vi "Vision Processing.vi"(4 "error in (no error)":errorcluster, 7 "Image Size":T1=enum."320x240") -> ()   [LabVIEW 2014]
uses:
  Vision Support Code/Camera Types.ctl
  <vilib>/Rock Robotics/WPI/Camera/WPI_CameraImageSize.ctl
  <vilib>/Rock Robotics/WPI/Camera/WPI_CameraWhite Balance Values.ctl
  <vilib>/Rock Robotics/WPI/Camera/WPI_CameraExposure Values.ctl
  <vilib>/Rock Robotics/WPI/Camera/WPI_CameraFrameRate.ctl
  Robot Global Data.vi
  <vilib>/vision/NI_Vision_Development_Module.lvlib
panel:
  in  "FPS":dbl
  out "Position_Debugger":i32
  in  "Right Boundary":dbl
  in  "Left Boundary":dbl
  out "Centering Command":enum16{"NULL", "RIGHT", "LEFT", "CENTER"}(ring)
  out "Horizontal Centering":dbl
  in  "Limit Tests?":bool
  in  "Camera Type":T2=enum."MS HD3000 square"
  in  "Aspect Fudge Factor":dbl=1.0
  out "Detected Totes":T3(array[cluster]) {"Normalized Rect"."Numeric 5" format="%#_2g"; "Normalized Rect"."Numeric 3" format="%#_2g"; "Normalized Rect"."Numeric 2" format="%#_2g"; "Normalized Rect"."Numeric" format="%#_2g"}
  in  "Score Threshold":dbl=75.0
  in  "Show Carpet Mask":bool
  in  "Carpet Color":T4(tab)
  in  "Red":T5={"Hue"={231.0, 14.0}, "Sat"={83.0, 255.0}, "Val"={52.5, 255.0}} {"Hue" scale=0.0..255.0 scale format="%#_3g"}
  in  "Blue":T5={"Hue"={119.0, 181.0}, "Sat"={33.0, 255.0}, "Val"={48.571428571428584, 255.0}} {"Hue" scale=0.0..255.0 scale format="%#_3g"}
  in  "Annotate":bool
  out "ms to process":u32
  out "Sorted Scores":T6(array[cluster]) {"Carpet" format="%#_3g"; "S" format="%#_3g"; "Trapezoid %" format="%#_3g"; "L" format="%#_3g"; "Area to CH" format="%#_3g"; "X" format="%#_3g"; "Y" format="%#_3g"}
  out "Particles":i32
  in  "Tote Color":T5={"Hue"={36.0, 50.923317529462665}, "Sat"={196.28571428571428, 255.0}, "Val"={163.92857142857144, 255.0}} {"Hue" scale=0.0..255.0 scale format="%#_3g"}
  out "Masked":T7(plugin-control)
  out "Original Image":T7(plugin-control)
  # "This is only the initial camera size.\nOther camera setup is done\non the diagram. Notice it is set\nonce before the loop but can be\nupdated within the loop if needed."
  # "Instructions:\nUse Source select image files from a directory or use a USB or IP camera connected to your laptop.\nUse Tote Color to threshold and build particles. Adjust calibration if needed.\nSelect which carpet color to use for scoring. Calibrate the colors if needed.\nAnnotations show the rectangle and the scores from top to bottom."
  # "Aspect Ratio"
  # "Density Profile"
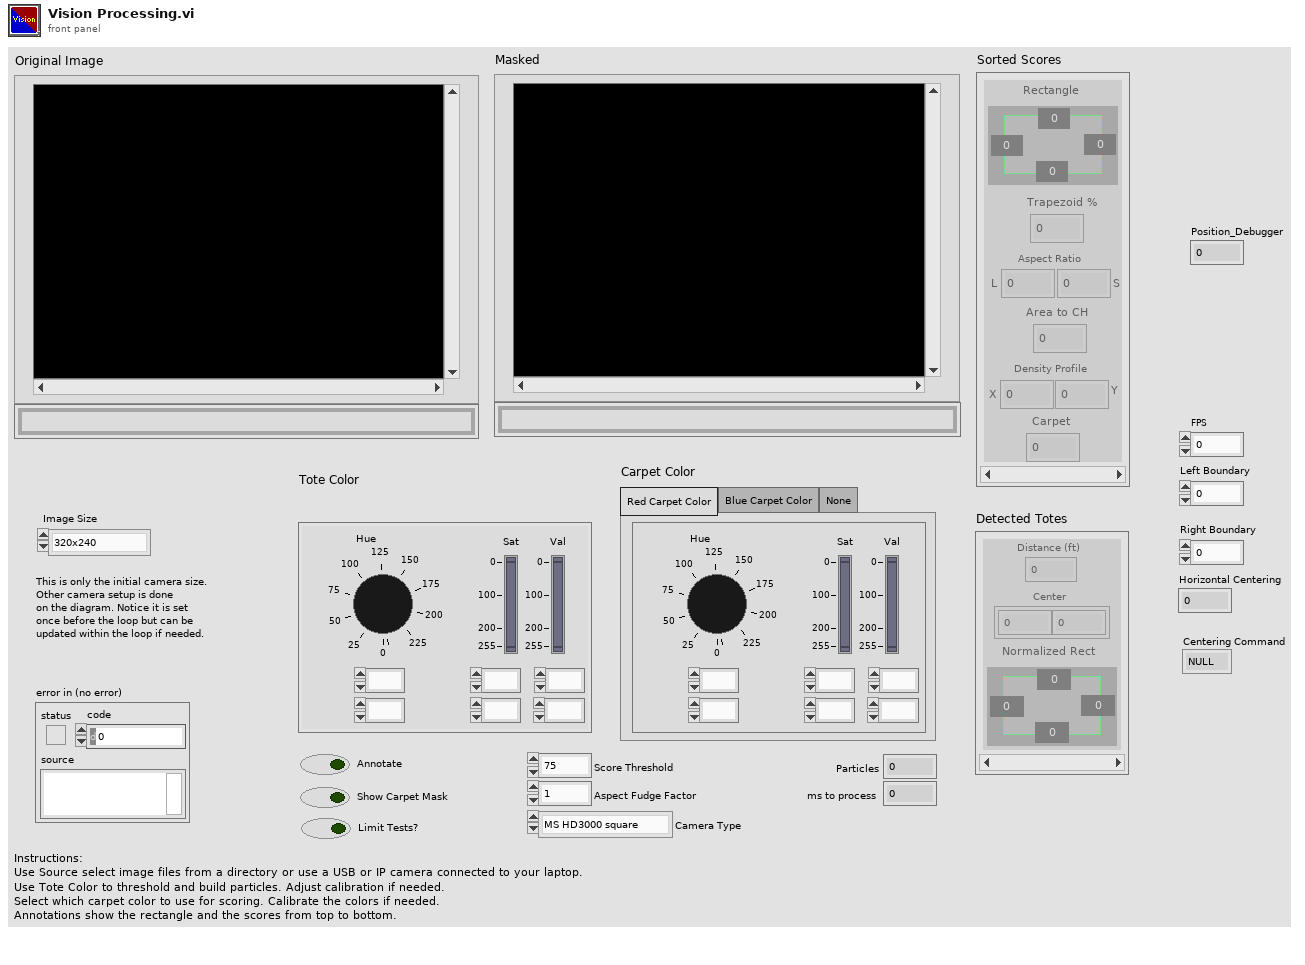
[diagram p1: front panel]
types:
  T1 = typedef "WPI_CameraImageSize.ctl" = enum16{"640x480", "320x240", "160x120", "Custom"}
  T2 = typedef "Camera Types.ctl" = enum16{"206", "1011", "1013", "MS HD3000 square", "MS HD3000 640x480"}
  T3 = cluster{"Distance (ft)":dbl, "Center":cluster{dbl, dbl}, "Normalized Rect":cluster{"Numeric":dbl, "Numeric 2":dbl, "Numeric 3":dbl, "Numeric 5":dbl}}[]
  T4 = enum32{"Red Carpet Color", "Blue Carpet Color", "None"}
  T5 = cluster{"Hue":cluster{dbl, dbl}, "Sat":cluster{dbl, dbl}, "Val":cluster{dbl, dbl}}
  T6 = cluster{"Rectangle":cluster{"Numeric":dbl, "Numeric 2":dbl, "Numeric 3":dbl, "Numeric 5":dbl}, "Trapezoid %":dbl, "L":dbl, "S":dbl, "Area to CH":dbl, "X":dbl, "Y":dbl, "Carpet":dbl}[]
  T7 = typedef "IMAQ Image.ctl" = refnum<image>
  T8 = typedef "WPI_CameraFrameRate.ctl" = u32
  T9 = typedef "WPI_CameraExposure Values.ctl" = enum16{"Auto", "Flicker-free 50 Hz", "Flicker-free 60 Hz", "Hold current", "Custom"}
  T10 = typedef "WPI_CameraWhite Balance Values.ctl" = enum16{"Auto", "Fixed indoor", "Fixed outdoor 1", "Fixed outdoor 2", "Fixed fluorescent 1", "Fixed fluorescent 2", "Hold current", "Custom"}
  T11 = typedef "Particle Parameters" = i32
  T12 = typedef "Image Type" = u32
  T13 = typedef "WPI_CameraDevRef.ctl" = cluster{"Camera Address":string, "CameraStatus":errorcluster}
  T14 = cluster{"Bounding box":cluster{"left":dbl, "top":dbl, "right":dbl, "bottom":dbl}, "Trapezoid":dbl, "Long Aspect":dbl, "Short Aspect":dbl, "Area to CH":dbl, "X Mask":dbl, "Y Mask":dbl, "Carpet":dbl}[]
  T15 = cluster{"Red":cluster{"Hue":cluster{dbl, dbl}, "Sat":cluster{dbl, dbl}, "Val":cluster{dbl, dbl}}, "Blue":cluster{"Hue":cluster{dbl, dbl}, "Sat":cluster{dbl, dbl}, "Val":cluster{dbl, dbl}}}
  T16 = cluster{cluster{"[0]":dbl, "[1]":dbl, "[2]":dbl, "[3]":dbl}, "Score":dbl, "Long Edge Score":dbl, "Short Edge Score":dbl, dbl, "X Score":dbl, "Y Score":dbl, "Carpet":dbl}[]
  T17 = cluster{"Found Totes[0]":cluster{"Distance (ft)":dbl, "Center":cluster{dbl, dbl}, "Normalized Rect":cluster{"Numeric":dbl, "Numeric 2":dbl, "Numeric 3":dbl, "Numeric 5":dbl}}, "Found Totes[1]":cluster{"Distance (ft)":dbl, "Center":cluster{dbl, dbl}, "Normalized Rect":cluster{"Numeric":dbl, "Numeric 2":dbl, "Numeric 3":dbl, "Numeric 5":dbl}}, "Found Totes[2]":cluster{"Distance (ft)":dbl, "Center":cluster{dbl, dbl}, "Normalized Rect":cluster{"Numeric":dbl, "Numeric 2":dbl, "Numeric 3":dbl, "Numeric 5":dbl}}, "Found Totes[3]":cluster{"Distance (ft)":dbl, "Center":cluster{dbl, dbl}, "Normalized Rect":cluster{"Numeric":dbl, "Numeric 2":dbl, "Numeric 3":dbl, "Numeric 5":dbl}}, "Found Totes[4]":cluster{"Distance (ft)":dbl, "Center":cluster{dbl, dbl}, "Normalized Rect":cluster{"Numeric":dbl, "Numeric 2":dbl, "Numeric 3":dbl, "Numeric 5":dbl}}, "Found Totes[5]":cluster{"Distance (ft)":dbl, "Center":cluster{dbl, dbl}, "Normalized Rect":cluster{"Numeric":dbl, "Numeric 2":dbl, "Numeric 3":dbl, "Numeric 5":dbl}}, "Found Totes[6]":cluster{"Distance (ft)":dbl, "Center":cluster{dbl, dbl}, "Normalized Rect":cluster{"Numeric":dbl, "Numeric 2":dbl, "Numeric 3":dbl, "Numeric 5":dbl}}, "Found Totes[7]":cluster{"Distance (ft)":dbl, "Center":cluster{dbl, dbl}, "Normalized Rect":cluster{"Numeric":dbl, "Numeric 2":dbl, "Numeric 3":dbl, "Numeric 5":dbl}}, "Found Totes[8]":cluster{"Distance (ft)":dbl, "Center":cluster{dbl, dbl}, "Normalized Rect":cluster{"Numeric":dbl, "Numeric 2":dbl, "Numeric 3":dbl, "Numeric 5":dbl}}}
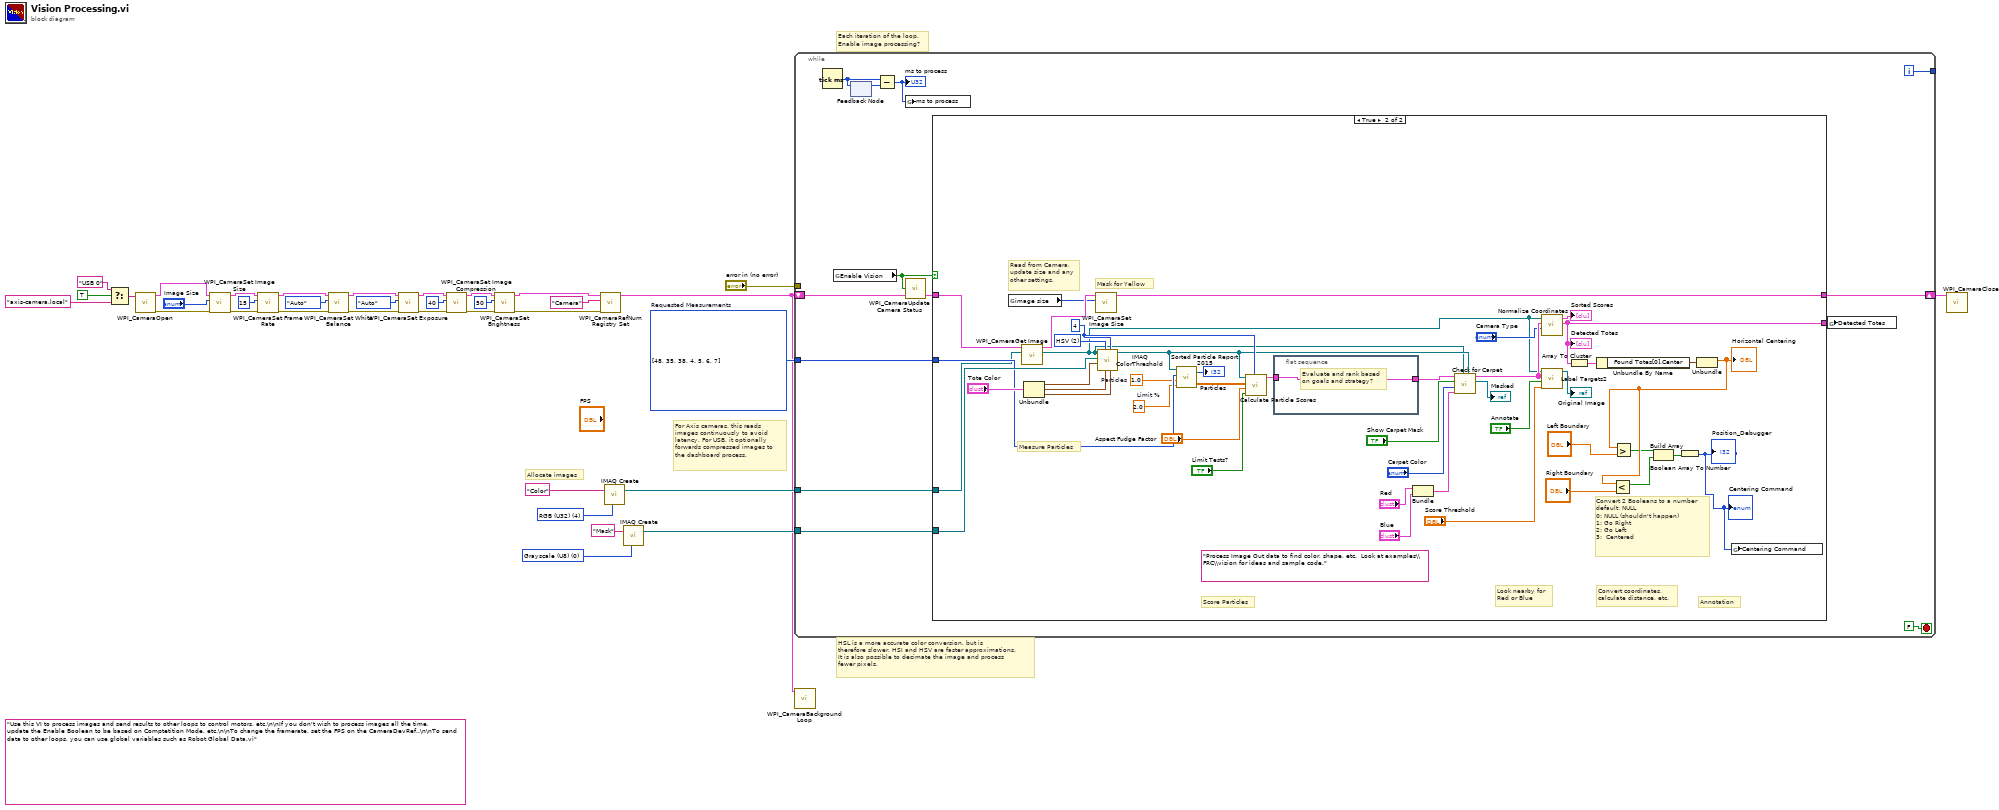
[diagram p0: block diagram]
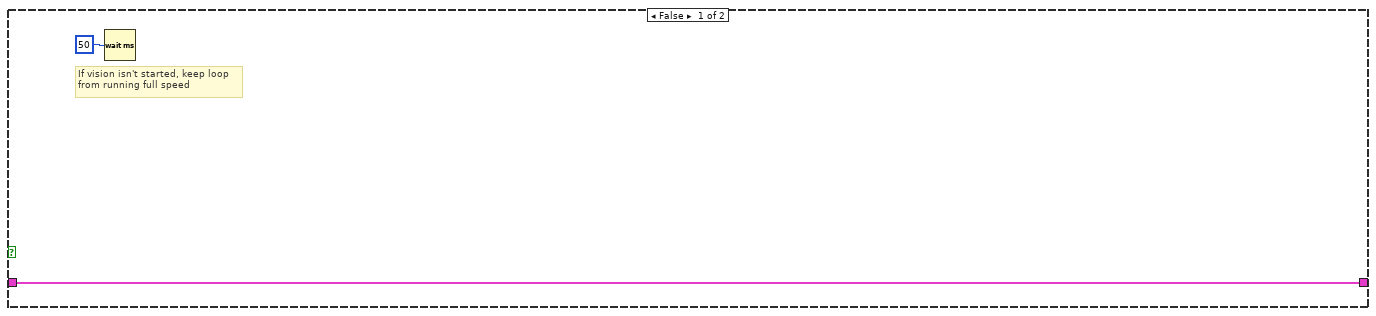
[diagram p2: hidden frame]
diagram:
  (unwired) "Use this VI to process images and send results to other loops to control motors, etc.\n\nIf you don't wish to process images all the time, update the Enable Boolean to be based on Comptetition Mode, etc.\n\nTo change the framerate, set the FPS on the CameraDevRef..\n\nTo send data to other loops, you can use global variables such as Robot Global Data.vi"
  w29 = T11[] [48, 35, 38, 4, 5, 6, 7] items=["Center of Mass X", "Center of Mass Y", "First Pixel X", "First Pixel Y", "Bounding Rect Left", "Bounding Rect Top", "Bounding Rect Right", "Bounding Rect Bottom", "Max Feret Diameter Start X", "Max Feret Diameter Start Y", "Max Feret Diameter End X", "Max Feret Diameter End Y", "Max Horiz. Segment Length Left", "Max Horiz. Segment Length Right", "Max Horiz. Segment Length Row", "-", "Bounding Rect Width", "Bounding Rect Height", "Bounding Rect Diagonal", "Perimeter", "Convex Hull Perimeter", "Holes' Perimeter", "Max Feret Diameter", "Equivalent Ellipse Major Axis", "Equivalent Ellipse Minor Axis", "Equivalent Ellipse Minor Axis (Feret)", "Equivalent Rect Long Side", "Equivalent Rect Short Side", "Equivalent Rect Diagonal", "Equivalent Rect Short Side (Feret)", "Average Horiz. Segment Length", "Average Vert. Segment Length", "Hydraulic Radius", "Waddel Disk Diameter", "-", "Area", "Holes' Area", "Particle & Holes' Area", "Convex Hull Area", "Image Area", "-", "Number of Holes", "Number of Horiz. Segments", "Number of Vert. Segments", "-", "Orientation", "Max Feret Diameter Orientation", "-", "% Area/Image Area", "% Area/(Particle & Holes' Area)", "Ratio of Equivalent Ellipse Axes", "Ratio of Equivalent Rect Sides", "-", "Elongation Factor", "Compactness Factor", "Heywood Circularity Factor", "Type Factor", "-", "Sum X", "Sum Y", "Sum XX", "Sum XY", "Sum YY", "Sum XXX", "Sum XXY", "Sum XYY", "Sum YYY", "-", "Moment of Inertia XX", "Moment of Inertia XY", "Moment of Inertia YY", "Moment of Inertia XXX", "Moment of Inertia XXY", "Moment of Inertia XYY", "Moment of Inertia YYY", "Norm. Moment of Inertia XX", "Norm. Moment of Inertia XY", "Norm. Moment of Inertia YY", "Norm. Moment of Inertia XXX", "Norm. Moment of Inertia XXY", "Norm. Moment of Inertia XYY", "Norm. Moment of Inertia YYY", "Hu Moment 1", "Hu Moment 2", "Hu Moment 3", "Hu Moment 4", "Hu Moment 5", "Hu Moment 6", "Hu Moment 7"]  # Requested Measurements
  w32 = T12 0 items=["Grayscale (U8)", "Grayscale (I16)", "Grayscale (SGL)", "Complex (CSG)", "RGB (U32)", "HSL (U32)", "RGB (U64)", "Grayscale (U16)"] ("Image Type")
  w34 = T12 4 items=["Grayscale (U8)", "Grayscale (I16)", "Grayscale (SGL)", "Complex (CSG)", "RGB (U32)", "HSL (U32)", "RGB (U64)", "Grayscale (U16)"] ("Image Type")
  # "Each iteration of the loop,\nEnable image processing?"
  # "HSL is a more accurate color conversion, but is\ntherefore slower. HSI and HSV are faster approximations.\nIt is also possible to decimate the image and process\nfewer pixels."
  # "For Axis cameras, this reads\nimages continuously to avoid\nlatency. For USB, it optionally\nforwards compressed images to\nthe dashboard process."
  # "Allocate images"
  n1 = Select(t="USB 0" ("format string"), s=TRUE ("dot notation? (F)"), f="axis-camera.local" ("format string")) -> (s? t:f=w28:string)
  n2 = call <vilib>:"WPI_CameraOpen.vi"("Camera Address"=w28) -> ("error out"=w15:errorcluster, "CameraDevRef"=w14:T13)  [unwired: 1 in, 8 out]
  n3 = call <vilib>:"WPI_CameraSet Image Size.vi"("error in (no error)"=w15, "Image Size"="Image Size", "CameraDevRef"=w14) -> ("error out"=w16:errorcluster, "CameraDevRef Out"=w13:T13)  [unwired: 1 in, 6 out]
  n4 = call <vilib>:"WPI_CameraSet Frame Rate.vi"("error in (no error)"=w16, "Frame Rate (fps)"=T8 15, "CameraDevRef"=w13) -> ("error out"=w17:errorcluster, "CameraDevRef Out"=w11:T13)  [unwired: 7 out]
  n5 = call <vilib>:"WPI_CameraSet White Balance.vi"("error in (no error)"=w17, "White Balance"=WPI_CameraWhite_Balance_Values."Auto", "CameraDevRef"=w11) -> ("error out"=w18:errorcluster, "CameraDevRef Out"=w12:T13)  [unwired: 1 in, 6 out]
  n6 = call <vilib>:"WPI_CameraSet Exposure.vi"("error in (no error)"=w18, "Exposure"=WPI_CameraExposure_Values."Auto", "CameraDevRef"=w12) -> ("error out"=w19:errorcluster, "CameraDevRef Out"=w9:T13)  [unwired: 1 in, 6 out]
  n7 = call <vilib>:"WPI_CameraSet Image Compression.vi"("error in (no error)"=w19, "Compression"=40, "CameraDevRef"=w9) -> ("error out"=w20:errorcluster, "CameraDevRef Out"=w10:T13)  [unwired: 7 out]
  n8 = call <vilib>:"WPI_CameraSet Brightness.vi"("error in (no error)"=w20, "Brightness"=50, "CameraDevRef"=w10) -> ("error out"=w22:errorcluster, "CameraDevRef Out"=w21:T13)  [unwired: 7 out]
  n9 = call <vilib>:"WPI_CameraRefNum Registry Set.vi"("error in (no error)"=w22, "refnum name"="Camera", "CameraDevRef"=w21) -> ("CameraDevRef"=w5:T13)  [unwired: 8 out]
  n10 = call "IMAQ Create"("Image Name"="Color", "Image Type"=w34) -> ("New Image"=w33:T7)  [unwired: 2 in, 2 out]
  n11 = call "IMAQ Create"("Image Name"="Mask", "Image Type"=w32) -> ("New Image"=w30:T7)  [unwired: 2 in, 2 out]
  n12 = while {
    tunnel: w33 -> [w43]
    tunnel: w30 -> [w47]
    tunnel: w29 -> [w46]
    tunnel: "error in (no error)" -> [_]
    tunnel: [w42] -> _
    shift-right: [w38] -> w1
    shift-left: w5 -> [w40]
    i -> [w42]
    stop <- FALSE stop-if-true
    n13 = Tick Count (ms)() -> (millisecond timer value=w44:u32)
    n14 = global read "Robot Global Data.vi" "Enable Vision"() -> (w41:bool)
    n15 = feedback-in #1(w44) -> ()
    n16 = feedback #1() -> (w45:u32)  [unwired: 1 in]
    n17 = Subtract(x=w44, y=w45) -> (x-y=w37:u32)
    "ms to process" <- w37
    n18 = global write "Robot Global Data.vi" "ms to process"(w37) -> ()
    n19 = call <vilib>:"WPI_CameraUpdate Camera Status.vi"("CameraDevRef In"=w40, "Enable Vision"=w41) -> ("CameraDevRef Out"=w39:T13)  [unwired: 3 in]
    n20 = case shown="True" w41 {
      tunnel: w47 -> [_ w95]
      tunnel: w46 -> [_ w89]
      tunnel: w39 -> [w49 w69]
      tunnel: w43 -> [_ w68]
      tunnel: [w49 w64] -> w38
      tunnel: [_ w60] -> w36
      frame False {
        # "If vision isn't started, keep loop\nfrom running full speed"
        n21 = Wait (ms)(milliseconds to wait=u32 50) -> ()  [unwired: 1 out]
      }
      frame True {
        (unwired) "Process Image Out data to find color, shape, etc.  Look at examples\\FRC\\vision for ideas and sample code."
        w78 = 4 ("Replace Value")
        w85 = 2.0  # Limit %
        w88 = 1.0  # Particles
        w94 = u16 2 items=["RGB", "HSL", "HSV", "HSI"] ("Color Mode")
        # "Convert 2 Booleans to a number\ndefault: NULL\n0: NULL (shouldn't happen)\n1: Go Right\n2: Go Left\n3:  Centered"
        # "Read from Camera,\nupdate size and any\nother settings."
        # "Measure Particles"
        # "Convert coordinates,\ncalculate distance, etc."
        # "Annotation"
        # "Score Particles"
        # "Mask for Yellow"
        # "Look nearby for\nRed or Blue"
        n22 = global read "Robot Global Data.vi" "image size"() -> (w65:T1)
        n23 = call <vilib>:"WPI_CameraGet Image.vi"("Image"=w68, "CameraDevRef"=w69) -> ("Image Out"=w67:T7, "CameraDevRef Out"=w66:T13)  [unwired: 7 in, 1 out]
        n24 = Unbundle("Tote Color") -> ("Hue"=w93:cluster{dbl, dbl}, "Sat"=w92:cluster{dbl, dbl}, "Val"=w91:cluster{dbl, dbl})
        n25 = call <vilib>:"WPI_CameraSet Image Size.vi"("Image Size"=w65, "CameraDevRef"=w66) -> ("CameraDevRef Out"=w64:T13)  [unwired: 2 in, 7 out]
        n26 = call "IMAQ ColorThreshold"("Blue or Luma or Val or Inten Range"=w91, "Replace Value"=w78, "Green or Sat Range"=w92, "Color Mode"=w94, "Red or Hue Range"=w93, "Image Dst"=w95, "Image Src"=w67) -> ("Image Dst Out"=w71:T7)  [unwired: 3 in, 1 out]
        n27 = call "Sorted Particle Report 2015.vi"("Min Area Size %"=w85, "Particle Count Limit"=w88, "Pixel Measurements"=w89, "Image in"=w71) -> ("Sorted Data"=w86:dbl[][], "Particles"=→"Particles":i32)
        n28 = call "Calculate Particle Scores.vi"("Pixel Value"=w78, "Limit Tests?"="Limit Tests?", "Aspect Fudge Factor"="Aspect Fudge Factor", "Sorted Data"=w86, "Image in"=w71) -> ("Scores"=w73:T14)  [unwired: 6 in]
        n29 = flat-sequence {
          tunnel: w73 -> [w96]
          tunnel: [w96] -> w72
          frame #0 {
            # "Evaluate and rank based\non goals and strategy?"
          }
        }
        n30 = Bundle("Red"="Red", "Blue"="Blue") -> (w79:T15)  [unwired: 1 in]
        n31 = call "Check for Carpet.vi"("Original Mask"=w71, "Original Color"=w67, "Carpet Colors"=w79, "Carpet Selector"="Carpet Color", "Combine Carpet Mask"="Show Carpet Mask", "Initial Scores"=w72) -> ("Updated Mask"=→"Masked":T7, "Updated Scores"=w77:T16)  [unwired: 4 in]
        n32 = call "Normalize Coordinates.vi"("Camera Type"="Camera Type", "Targets"=w77, "Image in"=w67) -> ("Found Totes"=w60:T3, "Sorted Scores"=→"Sorted Scores":T6)  [unwired: 7 in]
        "Detected Totes" <- w60
        n33 = call "Label Targets2.vi"("Score Threshold"="Score Threshold", "Annotate"="Annotate", "Targets"=w77, "Image in"=w67) -> ("Image out"=→"Original Image":T7)  [unwired: 7 in]
        n34 = Array To Cluster(array=w60) -> (cluster=w59:T17)
        n35 = Unbundle By Name(w59) -> ("Found Totes[0].Center"=w58:cluster{dbl, dbl})
        n36 = Unbundle(w58) -> (w55:dbl)  [unwired: 1 out]
        "Horizontal Centering" <- w55
        n37 = Less?(x=w55, y="Right Boundary") -> (x < y?=w53:bool)
        n38 = Greater?(x=w55, y="Left Boundary") -> (0:w54:bool)
        n39 = Build Array(w54, w53) -> (w52:bool[])
        n40 = Boolean Array To Number(Boolean array=w52) -> (number=w51:u32)
        "Centering Command" <- w51
        "Position_Debugger" <- w51
        n41 = global write "Robot Global Data.vi" "Centering Command"(w51) -> ()
      }
    }
    n42 = global write "Robot Global Data.vi" "Detected Totes"(w36) -> ()
  }
  n43 = call <vilib>:"WPI_CameraBackground Loop.vi"("CameraDevRef"=w5) -> ()  [unwired: 11 in]
  n44 = call <vilib>:"WPI_CameraClose.vi"("CameraDevRef"=w1) -> ()  [unwired: 1 in, 10 out]
